vi "simulate_P.vi"(4 "F_O":dbl caption="L/m", 6 "F_I":dbl=100.0 caption="L/m", 7 "V":dbl=1000.0 caption="L", 8 "dt":dbl=100.0 caption="sec", 11 "P_in":dbl) -> (3 "P_out":dbl)   [LabVIEW 2019]
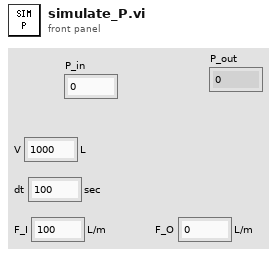
[diagram p1: front panel]
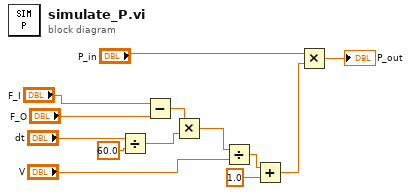
[diagram p0: block diagram]
diagram:
  n1 = Divide(x="dt", y=60.0) -> (x/y=w8:dbl)
  n2 = Subtract(x="F_I", y="F_O") -> (x-y=w9:dbl)
  n3 = Multiply(x=w9, y=w8) -> (x*y=w7:dbl)
  n4 = Divide(x=w7, y="V") -> (x/y=w5:dbl)
  n5 = Add(x=w5, y=1.0) -> (x+y=w2:dbl)
  n6 = Multiply(x="P_in", y=w2) -> (x*y=→"P_out":dbl)
